vi "getMode.vi"(8 "error in (no error)":errorcluster, 11 "PixelflySettings in":refnum<class "PixelflySettings.lvclass">) -> (0 "error out":errorcluster, 2 "mode":u16(ring)=2 items=["Asynch shutter", "Double shot", "Video mode", "Auto exposure"], 3 "PixelflySettings out":refnum<class "PixelflySettings.lvclass">)   [LabVIEW 2011, in "Tools.lvlib" / "Settings.lvlib" / "PixelflySettings.lvclass"]
uses:
  PixelflySettings.lvclass
  PixelflySettings.lvclass/PixelflySettings.ctl
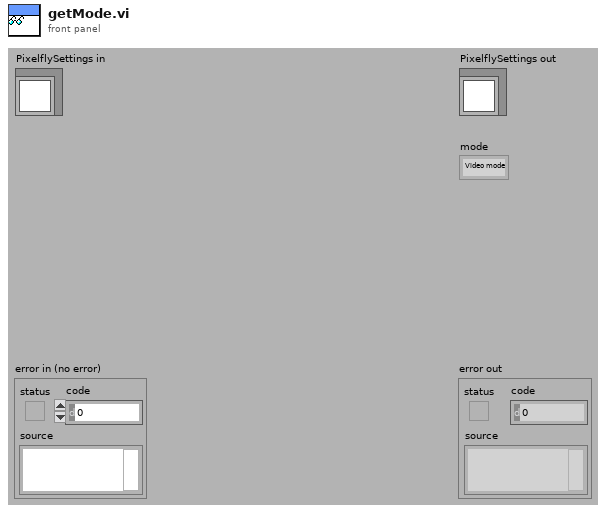
[diagram p1: front panel]
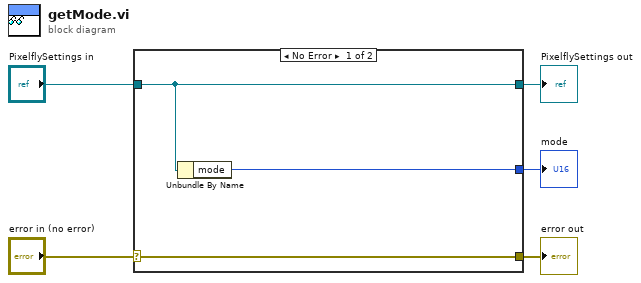
[diagram p0: block diagram]
diagram:
  n1 = case shown="No Error" "error in (no error)" {
    selector: "error in (no error)" -> [w8 w9]
    tunnel: [w8 w9] -> w4
    tunnel: [w7 w10] -> w2
    tunnel: "PixelflySettings in" -> [w7 w10]
    tunnel: [w6 _] -> w1
    frame No Error {
      n2 = Unbundle By Name(w7) -> ("mode"=w6:u16)
    }
    frame Error {
    }
  }
  "error out" <- w4
  "PixelflySettings out" <- w2
  "mode" <- w1
